vi "FRCts20_WebMethods_Redirect_Search.vi"(8 "error in (no error)":errorcluster, 9 "Team Index":u32, 10 "Status":string, 11 "httpRequestID":u32) -> (0 "error out":errorcluster, 3 "httpRequestID out":u32)   [LabVIEW 2013, in "FRCts20_WebMethods.lvlib"]
uses:
  FRCts20_WebMethods.lvlib
  <vilib>/wsapi/NI_WebServices.lvlib
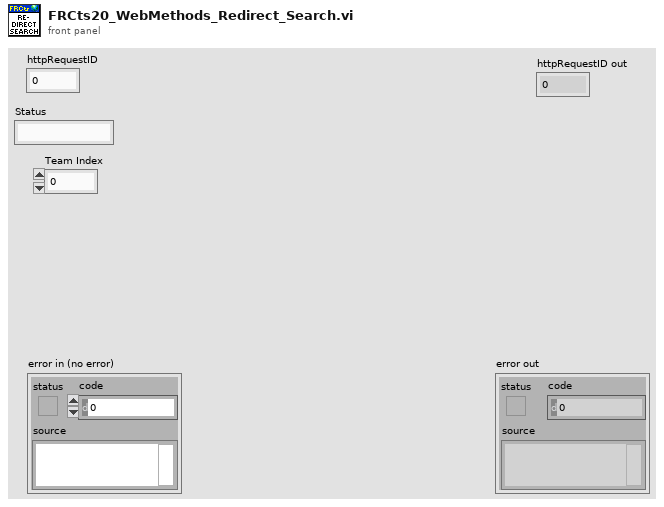
[diagram p1: front panel]
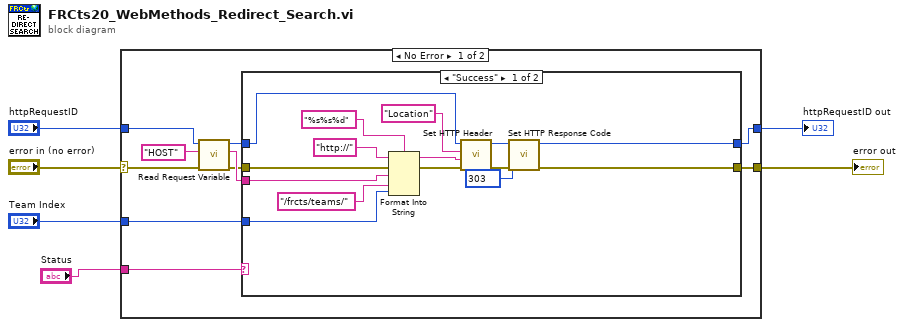
[diagram p0: block diagram]
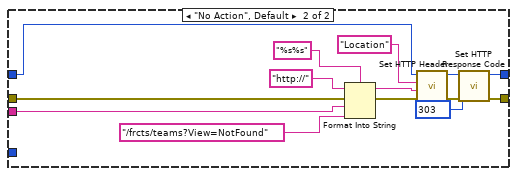
[diagram p2: hidden frame]
diagram:
  n1 = case shown="No Error" "error in (no error)" {
    selector: "error in (no error)" -> [w15 w47]
    tunnel: [w12 w47] -> w6
    tunnel: "httpRequestID" -> [w9 w46]
    tunnel: [w13 w46] -> w4
    tunnel: "Team Index" -> [w16 _]
    tunnel: "Status" -> [w7 _]
    frame No Error {
      n2 = call <vilib>:"Read Request Variable.vi"("error in (no error)"=w15, "variable name"="HOST", "httpRequestID"=w9) -> ("error out"=w10:errorcluster, "value"=w11:string, "httpRequestID out"=w8:u32)  [unwired: 6 in]
      n3 = case shown="\"Success\"" w7 {
        tunnel: w16 -> [w18 _]
        tunnel: [w28 w41] -> w13
        tunnel: [w27 w42] -> w12
        tunnel: w11 -> [w23 w36]
        tunnel: w10 -> [w22 w37]
        tunnel: w8 -> [w19 w33]
        frame "Success" {
          w17 = 303 items=["100"=100, "101"=101, "200"=200, "201"=201, "202"=202, "203"=203, "204"=204, "205"=205, "206"=206, "300"=300, "301"=301, "302"=302, "303"=303, "304"=304, "305"=305, "306"=306, "307"=307, "400"=400, "401"=401, "402"=402, "403"=403, "404"=404, "405"=405, "406"=406, "407"=407, "408"=408, "409"=409, "410"=410, "411"=411, "412"=412, "413"=413, "414"=414, "415"=415, "416"=416, "417"=417, "500"=500, "501"=501, "502"=502, "503"=503, "504"=504, "505"=505] ("response code (200)")
          n4 = Format Into String(format string="%s%s%d", initial string="http://", error in=w22, w23, "/frcts/teams/", w18) -> (resulting string=w20:string, error out=w21:errorcluster)
          n5 = call <vilib>:"Set HTTP Header.vi"("error in (no error)"=w21, "header value"=w20, "header"="Location", "httpRequestID"=w19) -> ("error out"=w30:errorcluster, "httpRequestID out"=w29:u32)  [unwired: 6 in]
          n6 = call <vilib>:"Set HTTP Response Code.vi"("error in (no error)"=w30, "response code (200)"=w17, "httpRequestID"=w29) -> ("error out"=w27:errorcluster, "httpRequestID out"=w28:u32)  [unwired: 7 in]
        }
        frame "No Action", Default {
          w32 = 303 items=["100"=100, "101"=101, "200"=200, "201"=201, "202"=202, "203"=203, "204"=204, "205"=205, "206"=206, "300"=300, "301"=301, "302"=302, "303"=303, "304"=304, "305"=305, "306"=306, "307"=307, "400"=400, "401"=401, "402"=402, "403"=403, "404"=404, "405"=405, "406"=406, "407"=407, "408"=408, "409"=409, "410"=410, "411"=411, "412"=412, "413"=413, "414"=414, "415"=415, "416"=416, "417"=417, "500"=500, "501"=501, "502"=502, "503"=503, "504"=504, "505"=505] ("response code (200)")
          n7 = Format Into String(format string="%s%s", initial string="http://", error in=w37, w36, "/frcts/teams?View=NotFound") -> (resulting string=w34:string, error out=w35:errorcluster)
          n8 = call <vilib>:"Set HTTP Header.vi"("error in (no error)"=w35, "header value"=w34, "header"="Location", "httpRequestID"=w33) -> ("error out"=w44:errorcluster, "httpRequestID out"=w43:u32)  [unwired: 6 in]
          n9 = call <vilib>:"Set HTTP Response Code.vi"("error in (no error)"=w44, "response code (200)"=w32, "httpRequestID"=w43) -> ("error out"=w42:errorcluster, "httpRequestID out"=w41:u32)  [unwired: 7 in]
        }
      }
    }
    frame Error {
    }
  }
  "error out" <- w6
  "httpRequestID out" <- w4
